vi "校准任务流程.vi"(9 "校准任务":T1[](array[typedef]), 10 "精度":dbl=4.0, 11 "模型":enum32{"线性", "多项式", "折线"}(ring)) -> ()   [LabVIEW 2016, in "斯坦道CODMn新电路板.lvlib"]
uses:
  <userlib>/_OpenG.lib/array/array.llb/Remove Duplicates from 1D Array (U16)__ogtk.vi
panel:
  out "元素":T1
  out "执行列表":T2(ring)
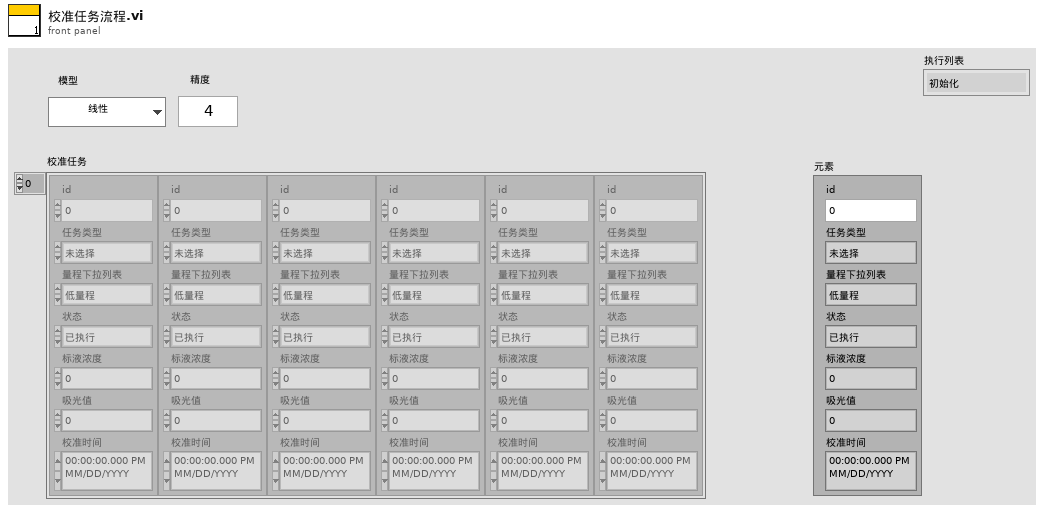
[diagram p1: front panel]
types:
  T1 = typedef "校准任务.ctl" = cluster{"id":u16, "任务类型":enum16{"未选择", "空白校准", "标样校准", "标样核查", "零点核查", "跨度核查"}, "量程下拉列表":enum16{"低量程", "高量程"}, "状态":enum16{"已执行", "待执行", "执行中", "停止"}, "标液浓度":dbl, "吸光值":dbl, "校准时间":timestamp}
  T2 = enum16{"初始化", "解析数据", "判断任务类型", "执行测试任务", "等待测试任务完成", "获取测试数据", "任务结束判定", "计算公式", "结束"}
  T3 = cluster{"时间标识":timestamp, "设备":string, "日志信息":string, "流程参数":string}
  T4 = cluster{"站号":u16, "量程切换":enum32{"H", "L", "AUTO"}, "控制命令":u16, "模式设置":enum16{"待机", "连续模式", "周期模式", "定点模式", "受控模式", "手动模式"}, "测量间隔":u16}
  T5 = cluster{"标液浓度1":dbl, "测量吸光度1":dbl, "样品1启用":bool, "标液浓度2":dbl, "测量吸光度2":dbl, "样品2启用":bool, "标液浓度3":dbl, "测量吸光度3":dbl, "样品3启用":bool, "标液浓度4":dbl, "测量吸光度4":dbl, "样品4启用":bool, "标液浓度5":dbl, "测量吸光度5":dbl, "样品5启用":bool, "模型":enum32{"线性", "多项式", "折线"}, "精度":dbl, "XY图":cluster{"X Values":dbl[], "Y Values":dbl[]}[], "拟合公式":string, "r^2":dbl, "标样一校准时间":timestamp, "标样二校准时间":timestamp, "标样三校准时间":timestamp, "标样四校准时间":timestamp, "标样五校准时间":timestamp, "二次方程":cluster{"x^2":dbl, "K":dbl, "B":dbl}, "标定时间":timestamp, "拟合公式 2":string, "r^2 2":dbl}
  T6 = enum16{"", "水样测量", "标样核查", "零点核查", "跨度核查", "空白测试", "平行样测试", "加标回收", "空白校准", "标样校准"}
  T7 = cluster{"因子编码":u32, "单位":u16, "标样参考值":sgl, "水样数据时间":timestamp, "水样实测值":sgl, "水样数据标识":string, "标样数据时间":timestamp, "标样实测值":sgl, "标样数据标识":string, "空白数据时间":timestamp, "空白实测值":sgl, "空白数据标识":string, "零点核查数据时间":timestamp, "零点核查实测值":sgl, "零点核查数据标识":string, "跨度核查数据时间":timestamp, "跨度核查实测值":sgl, "跨度核查数据标识":string, "加标回收数据时间":timestamp, "加标回收实测值":sgl, "加标回收数据标识":string, "平行样数据时间":timestamp, "平行样实测值":sgl, "平行样数据标识":string, "F0":sgl, "F1":sgl, "F2":sgl, "F3":sgl, "F4":sgl, "F5":sgl, "F6":sgl, "F7":sgl, "温度":sgl, "湿度":sgl, "X值":sgl, "fidrange":u16}
  T8 = cluster{"系统时间":timestamp, "工作状态":u16, "测量模式":enum16{"待机", "连续模式", "周期模式", "定点模式", "受控模式", "手动模式"}, "告警代码":u16, "故障代码":u16, "日志代码":u16, "软件版本":u16, "A":sgl, "B":sgl, "K":sgl, "当前滴定数":sgl, "T":sgl, "H":sgl, "id":u16, "flowid":u16, "量程":u16, "加热实时温度":sgl, "当前ORP值":sgl, "运行时间":sgl, "当前步骤剩余时间":sgl, "结束滴定数":sgl, "注射泵保温温度":sgl, "匹配滴定数X0":u16, "X^2":sgl, "X":sgl, "B 2":sgl}
  T9 = enum16{"未选择", "空白校准", "标样校准", "标样核查", "零点核查", "跨度核查"}
  T10 = cluster{"标液浓度1":dbl, "测量吸光度1":dbl, "样品1启用":bool, "标液浓度2":dbl, "测量吸光度2":dbl, "样品2启用":bool, "标液浓度3":dbl, "测量吸光度3":dbl, "样品3启用":bool, "标液浓度4":dbl, "测量吸光度4":dbl, "样品4启用":bool, "标液浓度5":dbl, "测量吸光度5":dbl, "样品5启用":bool, "模型":enum32{"线性", "多项式", "折线"}, "精度":dbl, "XY图":cluster{"X Values":dbl[], "Y Values":dbl[]}[], "拟合公式":string, "r^2":dbl, "标样一校准时间":timestamp, "标样二校准时间":timestamp, "标样三校准时间":timestamp, "标样四校准时间":timestamp, "标样五校准时间":timestamp, "二次方程":cluster{"c":dbl, "x":dbl, "x^2":dbl}, "标定时间":timestamp, "拟合公式 2":string, "r^2 2":dbl}[][]
  T11 = cluster{"标液浓度1":dbl, "测量吸光度1":dbl, "样品1启用":bool, "标液浓度2":dbl, "测量吸光度2":dbl, "样品2启用":bool, "标液浓度3":dbl, "测量吸光度3":dbl, "样品3启用":bool, "标液浓度4":dbl, "测量吸光度4":dbl, "样品4启用":bool, "标液浓度5":dbl, "测量吸光度5":dbl, "样品5启用":bool, "模型":enum32{"线性", "多项式", "折线"}, "精度":dbl, "XY图":cluster{"X Values":dbl[], "Y Values":dbl[]}[], "拟合公式":string, "r^2":dbl, "标样一校准时间":timestamp, "标样二校准时间":timestamp, "标样三校准时间":timestamp, "标样四校准时间":timestamp, "标样五校准时间":timestamp, "二次方程":cluster{"c":dbl, "x":dbl, "x^2":dbl}, "标定时间":timestamp, "拟合公式 2":string, "r^2 2":dbl}
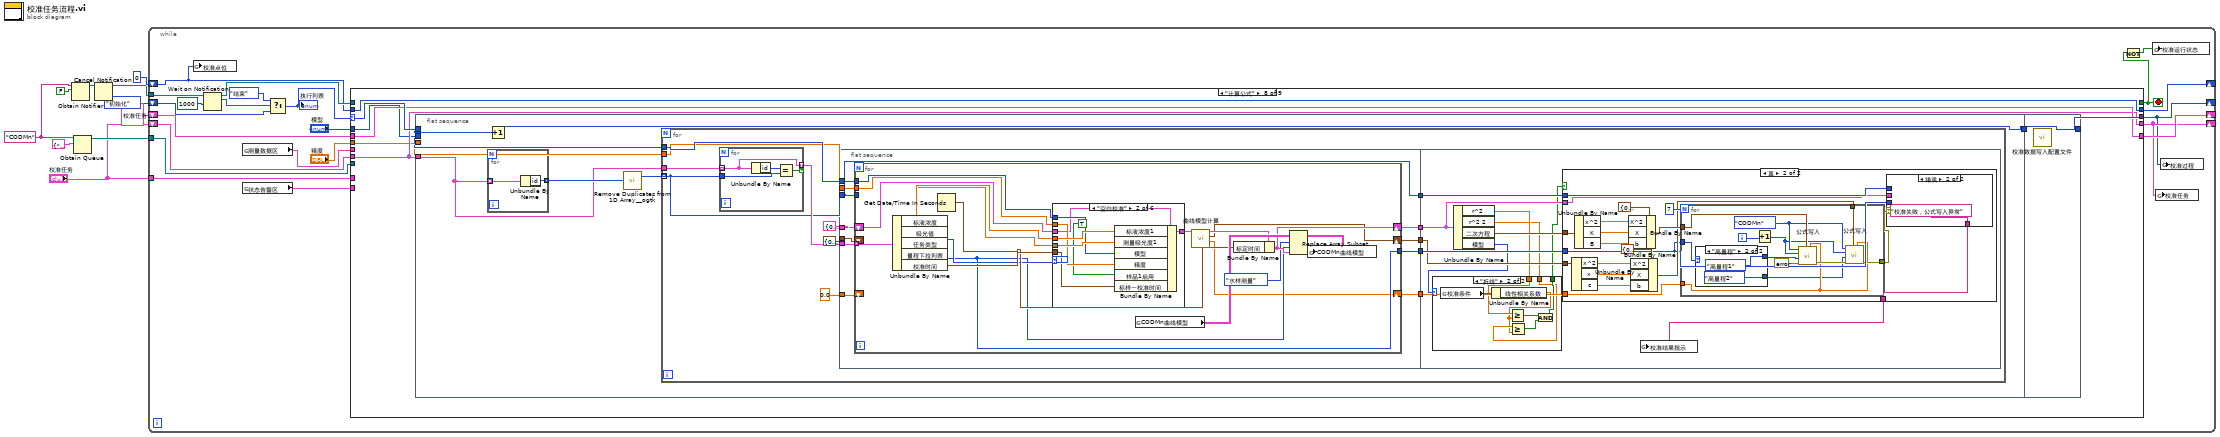
[diagram p0: block diagram]
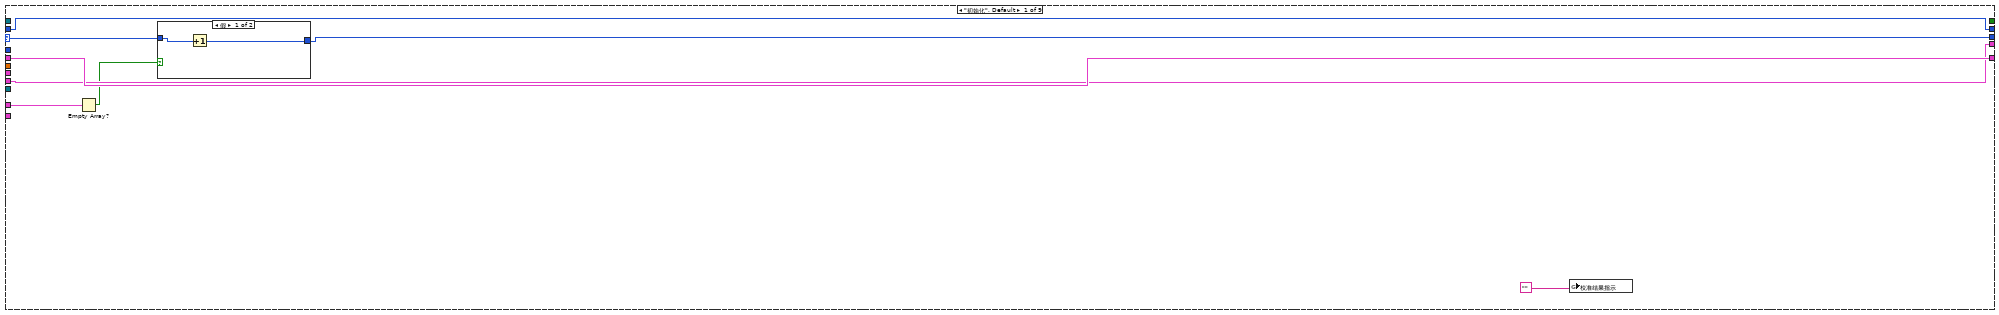
[diagram p2: hidden frame]
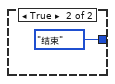
[diagram p3: hidden frame]
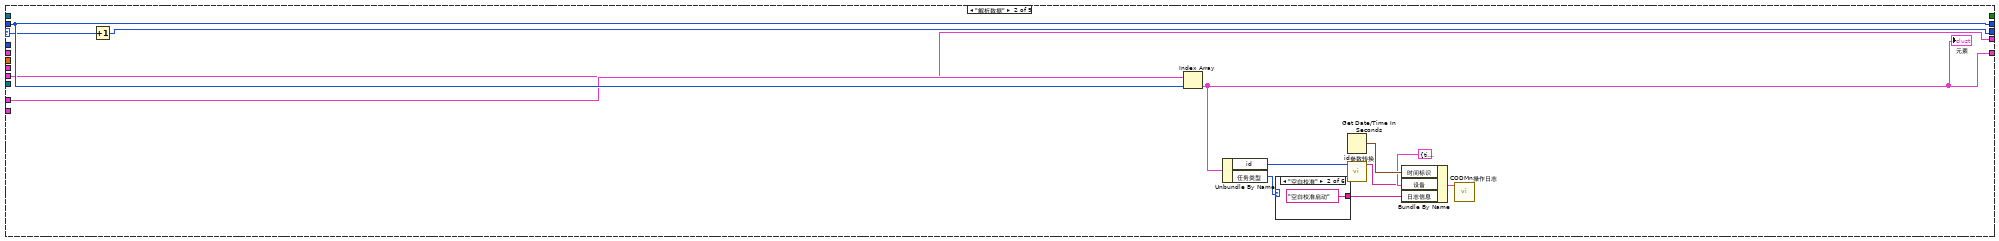
[diagram p4: hidden frame]
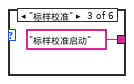
[diagram p6: hidden frame]
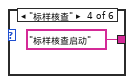
[diagram p7: hidden frame]
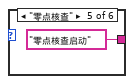
[diagram p8: hidden frame]
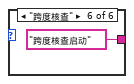
[diagram p9: hidden frame]
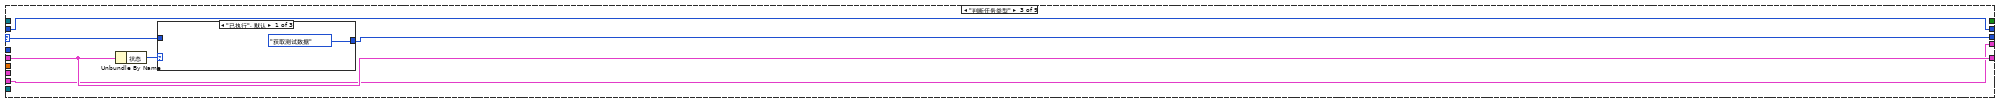
[diagram p10: hidden frame]
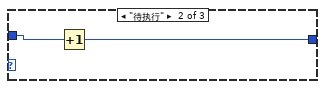
[diagram p11: hidden frame]
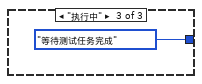
[diagram p12: hidden frame]
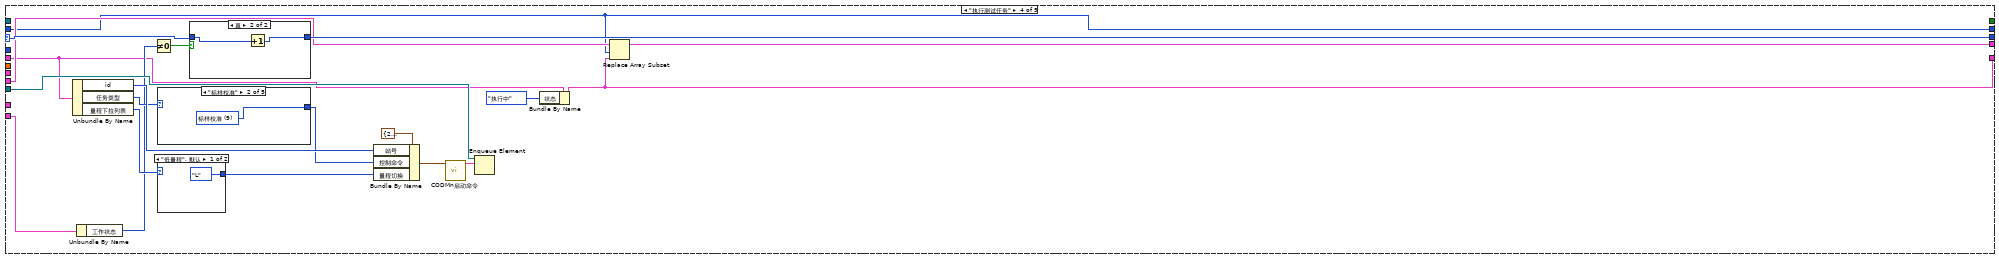
[diagram p13: hidden frame]
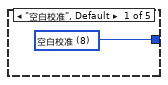
[diagram p15: hidden frame]
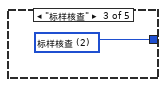
[diagram p16: hidden frame]
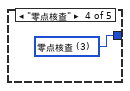
[diagram p17: hidden frame]
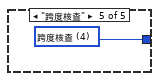
[diagram p18: hidden frame]
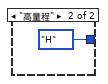
[diagram p19: hidden frame]
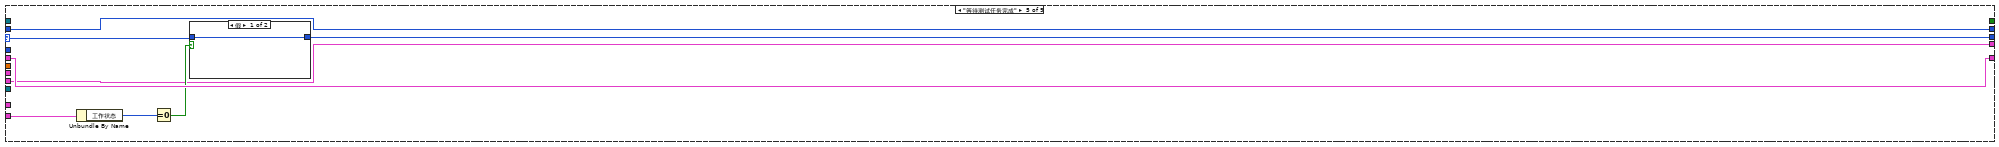
[diagram p20: hidden frame]
diagram:
  w2 = "CODMn" ("名称（未命名）")
  n1 = Obtain Notifier(name (unnamed)=w2, notification data type=FALSE) -> (notifier out=w5:refnum<notifier>)  [unwired: 2 in, 2 out]
  n2 = Obtain Queue(name (unnamed)=w2, element data type=cluster{"命令":string, "data":variant} {"命令"="", "data"=variant}) -> (queue out=w6:refnum<queue>)  [unwired: 3 in, 2 out]
  n3 = Cancel Notification(0:w5) -> (8:w4:refnum<notifier>)  [unwired: 1 in, 2 out]
  n4 = while {
    shift-right: [w12] -> _
    shift-left: 0 -> [w14]
    shift-right: [w32] -> _
    shift-left: T1 {"id"=0, "任务类型"=enum."未选择", "量程下拉列表"=enum."低量程", "状态"=enum."待执行", "标液浓度"=0.0, "吸光值"=0.0, "校准时间"=timestamp(0 s since 1904-01-01)} ("校准任务") -> [w31]
    shift-right: [w11] -> _
    shift-left: T2."初始化" ("执行列表") -> [w20]
    tunnel: w6 -> [w30]
    tunnel: w4 -> [w29]
    tunnel: "校准任务" -> [w26]
    shift-right: [w13] -> _
    shift-left: "校准任务" -> [w25]
    stop <- w15 stop-if-true
    n5 = global write "VARCODMn全局变量.vi" "校准点位"(w14) -> ()
    n6 = Wait on Notification(notifier=w29, timeout in ms (-1)=1000 ("超时毫秒(-1)")) -> (notifier out=w22:refnum<notifier>, notification=w21:bool)  [unwired: 2 in, 2 out]
    n7 = global read "VARCODMn全局变量.vi" "测量数据区"() -> (w27:T7)
    n8 = global read "VARCODMn全局变量.vi" "状态告警区"() -> (w28:T8)
    n9 = Select(t=T2."结束", s=w21, f=w20) -> (s? t:f=w19:T2)
    "执行列表" <- w19
    n10 = case shown="\"计算公式\"" w19 {
      selector: w19 -> [w38 w55 w64 w82 w105 w123 w160 w173 w345]
      tunnel: w14 -> [w39 w56 w66 w78 w108 w114 w161 w171 w343]
      tunnel: [w40 w47 w67 w75 w109 w118 w162 w170 w344] -> w32
      tunnel: w31 -> [w40 _ w67 w77 w109 w118 w162 w170 w344]
      tunnel: [w39 w56 w66 w78 w108 w114 w157 w171 w343] -> w12
      tunnel: [_ _ _ _ _ _ _ _ TRUE] -> w15
      tunnel: [w37 w54 w63 w81 w103 w122 w159 w172 w345] -> w11
      tunnel: w30 -> [_ _ _ w90 _ _ _ _ w340]
      tunnel: w22 -> [_ _ _ _ _ _ _ _ w339]
      tunnel: w28 -> [_ _ _ w85 w107 w113 _ _ _]
      tunnel: w27 -> [_ _ _ _ _ w125 _ _ _]
      tunnel: w26 -> [w35 w53 _ _ _ _ w158 _ _]
      tunnel: [w34 w52 w62 w79 w102 w120 w154 w169 w341] -> w13
      tunnel: w25 -> [w34 w52 w62 w80 w102 w119 w154 w169 w341]
      tunnel: "模型" -> [_ _ _ _ _ _ _ w168 _]
      tunnel: "精度" -> [_ _ _ _ _ _ _ w167 _]
      frame "初始化", Default {
        n11 = Empty Array?(array=w35) -> (empty?=w33:bool)
        n12 = case shown="假" w33 {
          tunnel: w38 -> [w42 _]
          tunnel: [w41 T2."结束"] -> w37
          frame False {
            n13 = Increment(x=w42) -> (x+1=w41:T2)
          }
          frame True {
          }
        }
        n14 = global write "VARCODMn全局变量.vi" "校准结果指示"("") -> ()
      }
      frame "解析数据" {
        n15 = Increment(x=w55) -> (x+1=w54:T2)
        n16 = Index Array(array=w53, index=w56) -> (element=w47:T1)
        "元素" <- w47
        n17 = Unbundle By Name(w47) -> ("id"=w46:u16, "任务类型"=w45:T9)
        n18 = case shown="\"空白校准\"" w45 {
          tunnel: [_ "空白校准启动" "标样校准启动" "标样核查启动" "零点核查启动" "跨度核查启动"] -> w44
          frame "未选择", Default {
          }
          frame "空白校准" {
          }
          frame "标样校准" {
          }
          frame "标样核查" {
          }
          frame "零点核查" {
          }
          frame "跨度核查" {
          }
        }
        n19 = Get Date/Time In Seconds() -> (seconds since 1Jan1904=w51:timestamp)
        n20 = call "id参数转换.vi"("id"=w46) -> ("table输出"=w48:string)  [unwired: 10 in]
        n21 = Bundle By Name(cluster=T3 {"时间标识"=timestamp(0 s since 1904-01-01), "设备"="", "日志信息"="", "流程参数"=""} ("data in"), "时间标识"=w51, "设备"=w48, "日志信息"=w44) -> (w50:T3)
        n22 = call "CODMn操作日志.vi"("data in"=w50) -> ()  [unwired: 11 in]
      }
      frame "判断任务类型" {
        n23 = Unbundle By Name(w67) -> ("状态"=w65:enum16{"已执行", "待执行", "执行中", "停止"})
        n24 = case shown="\"已执行\", 默认" w65 {
          tunnel: w64 -> [_ w70 _]
          tunnel: [T2."获取测试数据" w69 T2."等待测试任务完成"] -> w63
          frame "已执行", Default {
          }
          frame "待执行" {
            n25 = Increment(x=w70) -> (x+1=w69:T2)
          }
          frame "执行中" {
          }
        }
      }
      frame "执行测试任务" {
        n26 = Unbundle By Name(w77) -> ("id"=w89:u16, "任务类型"=w88:T9, "量程下拉列表"=w87:enum16{"低量程", "高量程"})
        n27 = Unbundle By Name(w85) -> ("工作状态"=w84:u16)
        n28 = Not Equal To 0?(x=w84) -> (x != 0?=w83:bool)
        n29 = case shown="\"标样校准\"" w88 {
          tunnel: [w95 w96 w97 w98 w99] -> w72
          frame "空白校准", Default {
            w95 = u16 8 items=["启动测量"=1, "标样核查"=2, "零点核查"=3, "跨度核查"=4, "空白测试"=5, "平行样测试"=6, "加标回收"=7, "空白校准"=8, "标样校准"=9, "初始化（清洗）"=10, "停止测试"=11, "仪器重启"=12, "校时"=13, "模式设置"=14, "测量间隔设置"=15, "调试"=22, "填充管路"=30, "清洗管路"=31, "清洗反应杯"=32] ("控制命令")
          }
          frame "标样校准" {
            w96 = u16 9 items=["启动测量"=1, "标样核查"=2, "零点核查"=3, "跨度核查"=4, "空白测试"=5, "平行样测试"=6, "加标回收"=7, "空白校准"=8, "标样校准"=9, "初始化（清洗）"=10, "停止测试"=11, "仪器重启"=12, "校时"=13, "模式设置"=14, "测量间隔设置"=15, "调试"=22, "填充管路"=30, "清洗管路"=31, "清洗反应杯"=32] ("控制命令")
          }
          frame "标样核查" {
            w97 = u16 2 items=["启动测量"=1, "标样核查"=2, "零点核查"=3, "跨度核查"=4, "空白测试"=5, "平行样测试"=6, "加标回收"=7, "空白校准"=8, "标样校准"=9, "初始化（清洗）"=10, "停止测试"=11, "仪器重启"=12, "校时"=13, "模式设置"=14, "测量间隔设置"=15, "调试"=22, "填充管路"=30, "清洗管路"=31, "清洗反应杯"=32] ("控制命令")
          }
          frame "零点核查" {
            w98 = u16 3 items=["启动测量"=1, "标样核查"=2, "零点核查"=3, "跨度核查"=4, "空白测试"=5, "平行样测试"=6, "加标回收"=7, "空白校准"=8, "标样校准"=9, "初始化（清洗）"=10, "停止测试"=11, "仪器重启"=12, "校时"=13, "模式设置"=14, "测量间隔设置"=15, "调试"=22, "填充管路"=30, "清洗管路"=31, "清洗反应杯"=32] ("控制命令")
          }
          frame "跨度核查" {
            w99 = u16 4 items=["启动测量"=1, "标样核查"=2, "零点核查"=3, "跨度核查"=4, "空白测试"=5, "平行样测试"=6, "加标回收"=7, "空白校准"=8, "标样校准"=9, "初始化（清洗）"=10, "停止测试"=11, "仪器重启"=12, "校时"=13, "模式设置"=14, "测量间隔设置"=15, "调试"=22, "填充管路"=30, "清洗管路"=31, "清洗反应杯"=32] ("控制命令")
          }
        }
        n30 = case shown="\"低量程\", 默认" w87 {
          tunnel: [enum32{"H", "L", "AUTO"}."L" ("量程切换") enum32{"H", "L", "AUTO"}."H" ("量程切换")] -> w86
          frame "低量程", Default {
          }
          frame "高量程" {
          }
        }
        n31 = case shown="真" w83 {
          tunnel: w82 -> [w92 w94]
          tunnel: [w92 w93] -> w81
          frame False {
          }
          frame True {
            n32 = Increment(x=w94) -> (x+1=w93:T2)
          }
        }
        n33 = Bundle By Name(cluster=T4 {"站号"=21, "量程切换"=enum."AUTO", "控制命令"=0, "模式设置"=enum."待机", "测量间隔"=0} ("参数"), "站号"=w89, "控制命令"=w72, "量程切换"=w86) -> (w73:T4)
        n34 = call "CODMn启动命令.vi"("参数"=w73) -> ("启动命令"=w91:cluster{"命令":string, "data":variant})  [unwired: 10 in]
        n35 = Enqueue Element(queue=w90, element=w91) -> ()  [unwired: 2 in, 3 out]
        n36 = Bundle By Name(cluster=w77, "状态"=enum16{"已执行", "待执行", "执行中", "停止"}."执行中") -> (w75:T1)
        n37 = Replace Array Subset(array=w80, new element=w75, index=w78) -> (w79:T1[])
      }
      frame "等待测试任务完成" {
        n38 = Unbundle By Name(w107) -> ("工作状态"=w106:u16)
        n39 = Equal To 0?(x=w106) -> (x = 0?=w104:bool)
        n40 = case shown="假" w104 {
          tunnel: w105 -> [w110 w112]
          tunnel: [w110 w111] -> w103
          frame False {
          }
          frame True {
            n41 = Increment(x=w112) -> (x+1=w111:T2)
          }
        }
      }
      frame "获取测试数据" {
        n42 = Unbundle By Name(w118) -> ("任务类型"=w124:T9, "状态"=w117:enum16{"已执行", "待执行", "执行中", "停止"})
        n43 = Increment(x=w123) -> (x+1=w122:T2)
        n44 = case shown="\"已执行\"" w117 {
          tunnel: w125 -> [_ w133]
          tunnel: w124 -> [_ w132]
          tunnel: [w126 w129] -> w121
          tunnel: w118 -> [w126 w128]
          tunnel: w113 -> [_ w127]
          frame "已执行" {
          }
          frame "待执行", Default {
            n45 = case shown="\"跨度核查\"" w132 {
              tunnel: w133 -> [w137 w141 w145 w149 w153]
              tunnel: [w136 w140 w144 w148 w152] -> w130
              tunnel: [w134 w138 w142 w146 w150] -> w131
              tunnel: w127 -> [w135 w139 w143 w147 w151]
              frame "空白校准", Default {
                n46 = Unbundle By Name(w135) -> ("匹配滴定数X0"=w134:u16)
                n47 = Unbundle By Name(w137) -> ("空白数据时间"=w136:timestamp)
              }
              frame "标样校准" {
                n48 = Unbundle By Name(w139) -> ("匹配滴定数X0"=w138:u16)
                n49 = Unbundle By Name(w141) -> ("标样数据时间"=w140:timestamp)
              }
              frame "标样核查" {
                n50 = Unbundle By Name(w143) -> ("匹配滴定数X0"=w142:u16)
                n51 = Unbundle By Name(w145) -> ("标样数据时间"=w144:timestamp)
              }
              frame "零点核查" {
                n52 = Unbundle By Name(w149) -> ("零点核查数据时间"=w148:timestamp)
                n53 = Unbundle By Name(w147) -> ("匹配滴定数X0"=w146:u16)
              }
              frame "跨度核查" {
                n54 = Unbundle By Name(w153) -> ("跨度核查数据时间"=w152:timestamp)
                n55 = Unbundle By Name(w151) -> ("匹配滴定数X0"=w150:u16)
              }
            }
            n56 = Bundle By Name(cluster=w128, "校准时间"=w130, "吸光值"=w131) -> (w129:T1)
          }
        }
        n57 = Bundle By Name(cluster=w121, "状态"=enum16{"已执行", "待执行", "执行中", "停止"}."已执行") -> (w115:T1)
        n58 = Replace Array Subset(array=w119, new element=w115, index=w114) -> (w120:T1[])
      }
      frame "任务结束判定" {
        n59 = Array Size(array=w158) -> (size(s)=w156:i32)
        n60 = Increment(x=w161) -> (x+1=w157:i32)
        n61 = Greater Or Equal?(x=w157, y=w156) -> (x >= y?=w155:bool)
        n62 = case shown="真" w155 {
          tunnel: w160 -> [_ w165]
          tunnel: [T2."解析数据" w164] -> w159
          frame False {
          }
          frame True {
            n63 = Increment(x=w165) -> (x+1=w164:T2)
          }
        }
      }
      frame "计算公式" {
        n64 = flat-sequence {
          tunnel: w173 -> [w180]
          tunnel: w169 -> [w176]
          tunnel: w168 -> [w175]
          tunnel: w167 -> [w174]
          tunnel: [w179] -> w166
          tunnel: [w338] -> w172
          tunnel: w166 -> [w338]
          frame #0 {
            n65 = for {
              tunnel: w176 -> [w337] mode=indexing
              tunnel: [w336] -> w178 mode=indexing
              n66 = Unbundle By Name(w337) -> ("id"=w336:u16)
            }
            n67 = Increment(x=w180) -> (x+1=w179:T2)
            n68 = call-poly <userlib>:"Remove Duplicates from 1D Array__ogtk.vi"("Input Array"=w178) -> ("Output Array"=w177:u16[])  [unwired: 1 out]
            n69 = for {
              tunnel: w177 -> [w191] mode=indexing
              tunnel: w176 -> [w193]
              tunnel: w175 -> [w190]
              tunnel: w174 -> [w189]
              n70 = for {
                tunnel: w193 -> [w333] mode=indexing
                tunnel: w191 -> [w335]
                tunnel: [w333] -> w192 mode=indexing if=w334
                n71 = Unbundle By Name(w333) -> ("id"=w332:u16)
                n72 = Equal?(x=w332, y=w335) -> (x = y?=w334:bool)
              }
              n73 = flat-sequence {
                tunnel: w192 -> [w204]
                tunnel: w191 -> [w199]
                tunnel: w190 -> [w203]
                tunnel: w189 -> [w202]
                tunnel: T5 {"标液浓度1"=0.0, "测量吸光度1"=0.0, "样品1启用"=FALSE, "标液浓度2"=0.0, "测量吸光度2"=0.0, "样品2启用"=FALSE, "标液浓度3"=0.0, "测量吸光度3"=0.0, "样品3启用"=FALSE, "标液浓度4"=0.0, "测量吸光度4"=0.0, "样品4启用"=FALSE, "标液浓度5"=0.0, "测量吸光度5"=0.0, "样品5启用"=FALSE, "模型"=enum."线性", "精度"=4.0, "XY图"=[], "拟合公式"="", "r^2"=0.0, "标样一校准时间"=timestamp(0 s since 1904-01-01), "标样二校准时间"=timestamp(0 s since 1904-01-01), "标样三校准时间"=timestamp(0 s since 1904-01-01), "标样四校准时间"=timestamp(0 s since 1904-01-01), "标样五校准时间"=timestamp(0 s since 1904-01-01), "二次方程"={"x^2"=0.0, "K"=0.0, "B"=0.0}, "标定时间"=timestamp(0 s since 1904-01-01), "拟合公式 2"="", "r^2 2"=0.0} ("曲线模型") -> [w201]
                tunnel: [w200] -> w188
                tunnel: [w199] -> w187
                tunnel: [w198] -> w186
                tunnel: [w197] -> w184
                tunnel: cluster{"c":dbl, "x":dbl, "x^2":dbl} {"c"=0.0, "x"=0.0, "x^2"=0.0} ("二次方程 2") -> [w196]
                tunnel: [w195] -> w182
                tunnel: 0.0 ("公式切换阈值滴定数(0~9999)") -> [w194]
                tunnel: w188 -> [w271]
                tunnel: w187 -> [w273]
                tunnel: w186 -> [w272]
                tunnel: w184 -> [w269]
                tunnel: w182 -> [w268]
                frame #0 {
                  n74 = for {
                    tunnel: w204 -> [w222] mode=indexing
                    tunnel: w199 -> [_]
                    tunnel: w203 -> [w219]
                    tunnel: w202 -> [w218]
                    shift-right: [w210] -> w200
                    shift-left: w201 -> [w217]
                    tunnel: [w208] -> w198
                    shift-right: [w207] -> w197
                    shift-left: w196 -> [_]
                    shift-right: [w206] -> w195
                    shift-left: w194 -> [_]
                    n75 = Unbundle By Name(w222) -> ("标液浓度"=w221:dbl, "吸光值"=w220:dbl, "任务类型"=w209:T9, "量程下拉列表"=w208:enum16{"低量程", "高量程"}, "校准时间"=w216:timestamp)
                    n76 = Get Date/Time In Seconds() -> (seconds since 1Jan1904=w212:timestamp)
                    n77 = case shown="\"空白校准\"" w209 {
                      tunnel: w221 -> [_ w231 w239 w247 w255 w263]
                      tunnel: w220 -> [_ w230 w232 w246 w254 w262]
                      tunnel: w219 -> [_ w229 w238 w245 w253 w261]
                      tunnel: w218 -> [_ w228 w237 w244 w252 w260]
                      tunnel: w217 -> [w223 w226 w235 w242 w250 w258]
                      tunnel: [w223 w224 w234 w241 w249 w257] -> w215
                      tunnel: w216 -> [_ w225 w233 w240 w248 w256]
                      frame "未选择", Default {
                        (unwired) T6."" ("测量模式")
                      }
                      frame "空白校准" {
                        n78 = Bundle By Name(cluster=w226, "标液浓度1"=w231, "测量吸光度1"=w230, "模型"=w229, "精度"=w228, "样品1启用"=TRUE, "标样一校准时间"=w225) -> (w224:T5)
                      }
                      frame "标样校准" {
                        (unwired) T6."标样校准" ("测量模式")
                        n79 = Bundle By Name(cluster=w235, "标液浓度2"=w239, "测量吸光度2"=w232, "模型"=w238, "精度"=w237, "样品2启用"=TRUE ("样品1启用"), "标样二校准时间"=w233) -> (w234:T5)
                      }
                      frame "标样核查" {
                        (unwired) T6."标样核查" ("测量模式")
                        n80 = Bundle By Name(cluster=w242, "标液浓度3"=w247, "测量吸光度3"=w246, "模型"=w245, "精度"=w244, "样品3启用"=TRUE ("样品1启用"), "标样三校准时间"=w240) -> (w241:T5)
                      }
                      frame "零点核查" {
                        (unwired) T6."零点核查" ("测量模式")
                        n81 = Bundle By Name(cluster=w250, "标液浓度4"=w255, "测量吸光度4"=w254, "模型"=w253, "精度"=w252, "样品4启用"=TRUE ("样品1启用"), "标样四校准时间"=w248) -> (w249:T5)
                      }
                      frame "跨度核查" {
                        (unwired) T6."跨度核查" ("测量模式")
                        n82 = Bundle By Name(cluster=w258, "标液浓度5"=w263, "测量吸光度5"=w262, "模型"=w261, "精度"=w260, "样品5启用"=TRUE ("样品1启用"), "标样五校准时间"=w256) -> (w257:T5)
                      }
                    }
                    n83 = global read "校准数据全局变量.vi" "CODMn曲线模型"() -> (w214:T10)
                    n84 = call "曲线模型计算.vi"("曲线模型"=w215) -> ("公式切换阈值滴定数(0~9999)"=w206:dbl, "二次方程 2"=w207:cluster{"c":dbl, "x":dbl, "x^2":dbl}, "输出簇"=w211:T11)  [unwired: 8 in]
                    n85 = Bundle By Name(cluster=w211, "标定时间"=w212) -> (w210:T11)
                    n86 = Replace Array Subset(array=w214, new element=w210, index (row)=T6."水样测量" ("测量模式"), index (col)=w208) -> (w213:T10)
                    n87 = global write "校准数据全局变量.vi" "CODMn曲线模型"(w213) -> ()
                  }
                }
                frame #1 {
                  n88 = Unbundle By Name(w271) -> ("r^2"=w266:dbl, "r^2 2"=w265:dbl, "二次方程"=w274:cluster{"x^2":dbl, "K":dbl, "B":dbl}, "模型"=w267:enum32{"线性", "多项式", "折线"})
                  n89 = case shown="\"折线\"" w267 {
                    tunnel: w266 -> [w276 w280]
                    tunnel: w265 -> [_ w281]
                    tunnel: [w277 w282] -> w264
                    frame "线性", Default {
                      n90 = global read "CODMn断电保存全局变量.vi" "校准条件"() -> (w278:cluster{"线性相关系数":dbl})
                      n91 = Unbundle By Name(w278) -> ("线性相关系数"=w275:dbl)
                      n92 = Greater Or Equal?(x=w276, y=w275) -> (x >= y?=w277:bool)
                    }
                    frame "折线" {
                      n93 = global read "CODMn断电保存全局变量.vi" "校准条件"() -> (w285:cluster{"线性相关系数":dbl})
                      n94 = Unbundle By Name(w285) -> ("线性相关系数"=w279:dbl)
                      n95 = Greater Or Equal?(x=w280, y=w279) -> (x >= y?=w284:bool)
                      n96 = Greater Or Equal?(x=w281, y=w279) -> (x >= y?=w283:bool)
                      n97 = And(x=w284, y=w283) -> (x .and. y?=w282:bool)
                    }
                  }
                  n98 = case shown="真" w264 {
                    tunnel: w274 -> [_ w306]
                    tunnel: w273 -> [w288 w305]
                    tunnel: w272 -> [_ w294]
                    tunnel: w271 -> [_ w304]
                    tunnel: [w286 w303] -> w270
                    tunnel: w269 -> [_ w302]
                    tunnel: w268 -> [_ w293]
                    frame False {
                      w286 = "校准失败，校准条件未满足" ("日志信息")
                      n99 = call "id参数转换.vi"("id"=w288) -> ("table输出"=w287:string)  [unwired: 10 in]
                      n100 = Get Date/Time In Seconds() -> (seconds since 1Jan1904=w291:timestamp)
                      n101 = Bundle By Name(cluster=T3 {"时间标识"=timestamp(0 s since 1904-01-01), "设备"="", "日志信息"="", "流程参数"=""} ("data in"), "时间标识"=w291, "设备"=w287, "日志信息"=w286) -> (w290:T3)
                      n102 = call "CODMn操作日志.vi"("data in"=w290) -> ()  [unwired: 11 in]
                    }
                    frame True {
                      n103 = Unbundle By Name(w302) -> ("x^2"=w298:dbl, "x"=w297:dbl, "c"=w296:dbl)
                      n104 = Unbundle By Name(w306) -> ("x^2"=w308:dbl, "K"=w309:dbl, "B"=w310:dbl)
                      n105 = Bundle By Name(cluster=cluster{"X^2":dbl, "X":dbl, "b":dbl} {"X^2"=0.0, "X"=0.0, "b"=0.0} ("公式"), "X^2"=w308, "X"=w309, "b"=w310) -> (w300:cluster{"X^2":dbl, "X":dbl, "b":dbl})
                      n106 = Bundle By Name(cluster=cluster{"X^2":dbl, "X":dbl, "b":dbl} {"X^2"=0.0, "X"=0.0, "b"=0.0} ("公式"), "X^2"=w298, "X"=w297, "b"=w296) -> (w295:cluster{"X^2":dbl, "X":dbl, "b":dbl})
                      n107 = for {
                        N: 7 -> [_]
                        tunnel: w300 -> [w321]
                        tunnel: [w319] -> w292
                        tunnel: w295 -> [w318]
                        tunnel: w293 -> [w317]
                        tunnel: w294 -> [w315]
                        i -> [w312]
                        w316 = enum16{"CODMn"}."CODMn" ("测量参数")
                        n108 = case shown="\"高量程\"" w315 {
                          tunnel: [enum16{"低量程1", "低量程2", "高量程1", "高量程2"}."低量程1" ("量程") enum16{"低量程1", "低量程2", "高量程1", "高量程2"}."高量程1" ("量程")] -> w314
                          tunnel: [enum16{"低量程1", "低量程2", "高量程1", "高量程2"}."低量程2" ("量程") enum16{"低量程1", "低量程2", "高量程1", "高量程2"}."高量程2" ("量程")] -> w313
                          frame "低量程", Default {
                          }
                          frame "高量程" {
                          }
                        }
                        n109 = Increment(x=w312) -> (x+1=w311:i32)
                        n110 = call "公式写入.vi"("临界滴定数"=w317, "公式"=w321, "error in (no error)"=errorcluster {"status"=FALSE, "code"=0, "source"=""} ("error out"), "量程"=w314, "测量模式"=w311, "测量参数"=w316) -> ("error out"=w320:errorcluster)  [unwired: 5 in]
                        n111 = call "公式写入.vi"("临界滴定数"=w317, "公式"=w318, "error in (no error)"=w320, "量程"=w313, "测量模式"=w311, "测量参数"=w316) -> ("error out"=w319:errorcluster)  [unwired: 5 in]
                      }
                      n112 = case shown="错误" w292 {
                        tunnel: w305 -> [w330 _]
                        tunnel: w294 -> [w329 _]
                        tunnel: w304 -> [w327 _]
                        tunnel: ["校准成功" "校准失败，公式写入异常"] -> w303
                        frame No Error {
                          n113 = call "校准记录.vi"("曲线模型"=w327, "量程"=w329, "校准参数"=w330) -> ()  [unwired: 8 in, 1 out]
                        }
                        frame Error {
                        }
                      }
                    }
                  }
                  n114 = global write "VARCODMn全局变量.vi" "校准结果指示"(w270) -> ()
                }
              }
            }
          }
          frame #1 {
            n115 = call "校准数据写入配置文件.vi"() -> ()  [unwired: 11 in, 1 out]
          }
        }
      }
      frame "结束" {
        n116 = Release Notifier(notifier=w339) -> ()  [unwired: 2 in, 3 out]
        n117 = Release Queue(queue=w340) -> ()  [unwired: 2 in, 3 out]
      }
    }
    n118 = Not(x=w15) -> (.not. x?=w16:bool)
    n119 = global write "VARCODMn全局变量.vi" "校准运行状态"(w16) -> ()
    n120 = global write "VARCODMn全局变量.vi" "校准任务"(w13) -> ()
    n121 = global write "VARCODMn全局变量.vi" "校准过程"(w11) -> ()
  }
